vi "Write Configuration File.vi"(8 "error in (no error)":errorcluster, 10 "User Config":T1={"Password"="admin", "cDAQ Name"="cDAQ9188-1A2B7A8"}, 11 "Filepath":path=path "C:/PAS Circulation Tester/Configuration/userConfig.txt") -> (0 "error out":errorcluster)   [LabVIEW 2014]
uses:
  User Configuration.ctl
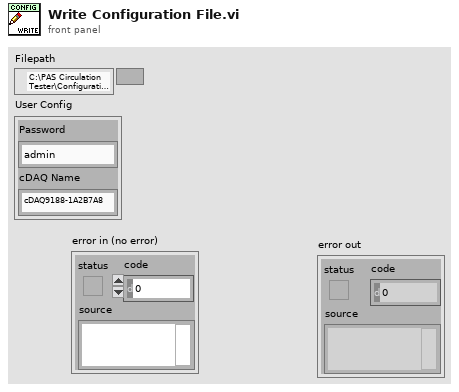
[diagram p1: front panel]
types:
  T1 = typedef "User Configuration.ctl" = cluster{"Password":string, "cDAQ Name":string}
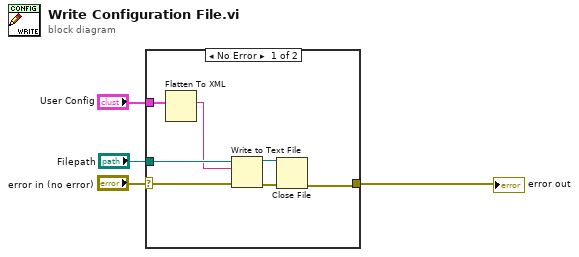
[diagram p0: block diagram]
diagram:
  n1 = case shown="No Error" "error in (no error)" {
    selector: "error in (no error)" -> [w11 w12]
    tunnel: [w5 w12] -> w4
    tunnel: "User Config" -> [w10 _]
    tunnel: "Filepath" -> [w9 _]
    frame No Error {
      n2 = Flatten To XML(anything=w10) -> (xml string=w8:string)
      n3 = Write to Text File(file (use dialog)=w9, text=w8, error in=w11) -> (refnum out=w6:refnum<file>, error out=w7:errorcluster)  [unwired: 1 in, 1 out]
      n4 = Close File(refnum=w6, error in=w7) -> (error out=w5:errorcluster)  [unwired: 1 out]
    }
    frame Error {
    }
  }
  "error out" <- w4
